vi "RT-Data-in.vi"(2 "cluster":T1, 3 "Amount of Inputs":i32) -> (0 "Error":T1, 1 "Bicep+Triceps":dbl[](array[numeric]))   [LabVIEW 2020]
uses:
  <vilib>/Utility/error.llb/Error Cluster From Error Code.vi
  <vilib>/rvi/errors/niLvFpgaAdjustHostInterfaceError.vi
  <vilib>/rvi/interface/nirviReadWriteControl/nirviReadWriteControl.xnode
  NiFpgaLv.dll
  <vilib>/rvi/interface/Simulation/niFpgaSimulationCallBeginRW.vi
panel:
  in  "Size of Window":i32=240
  out "BicepWindow":dbl[](array[numeric])
  out "TricepWindow":dbl[](array[numeric])
  out "data 5":dbl(graph)
  out "data 4":dbl(graph)
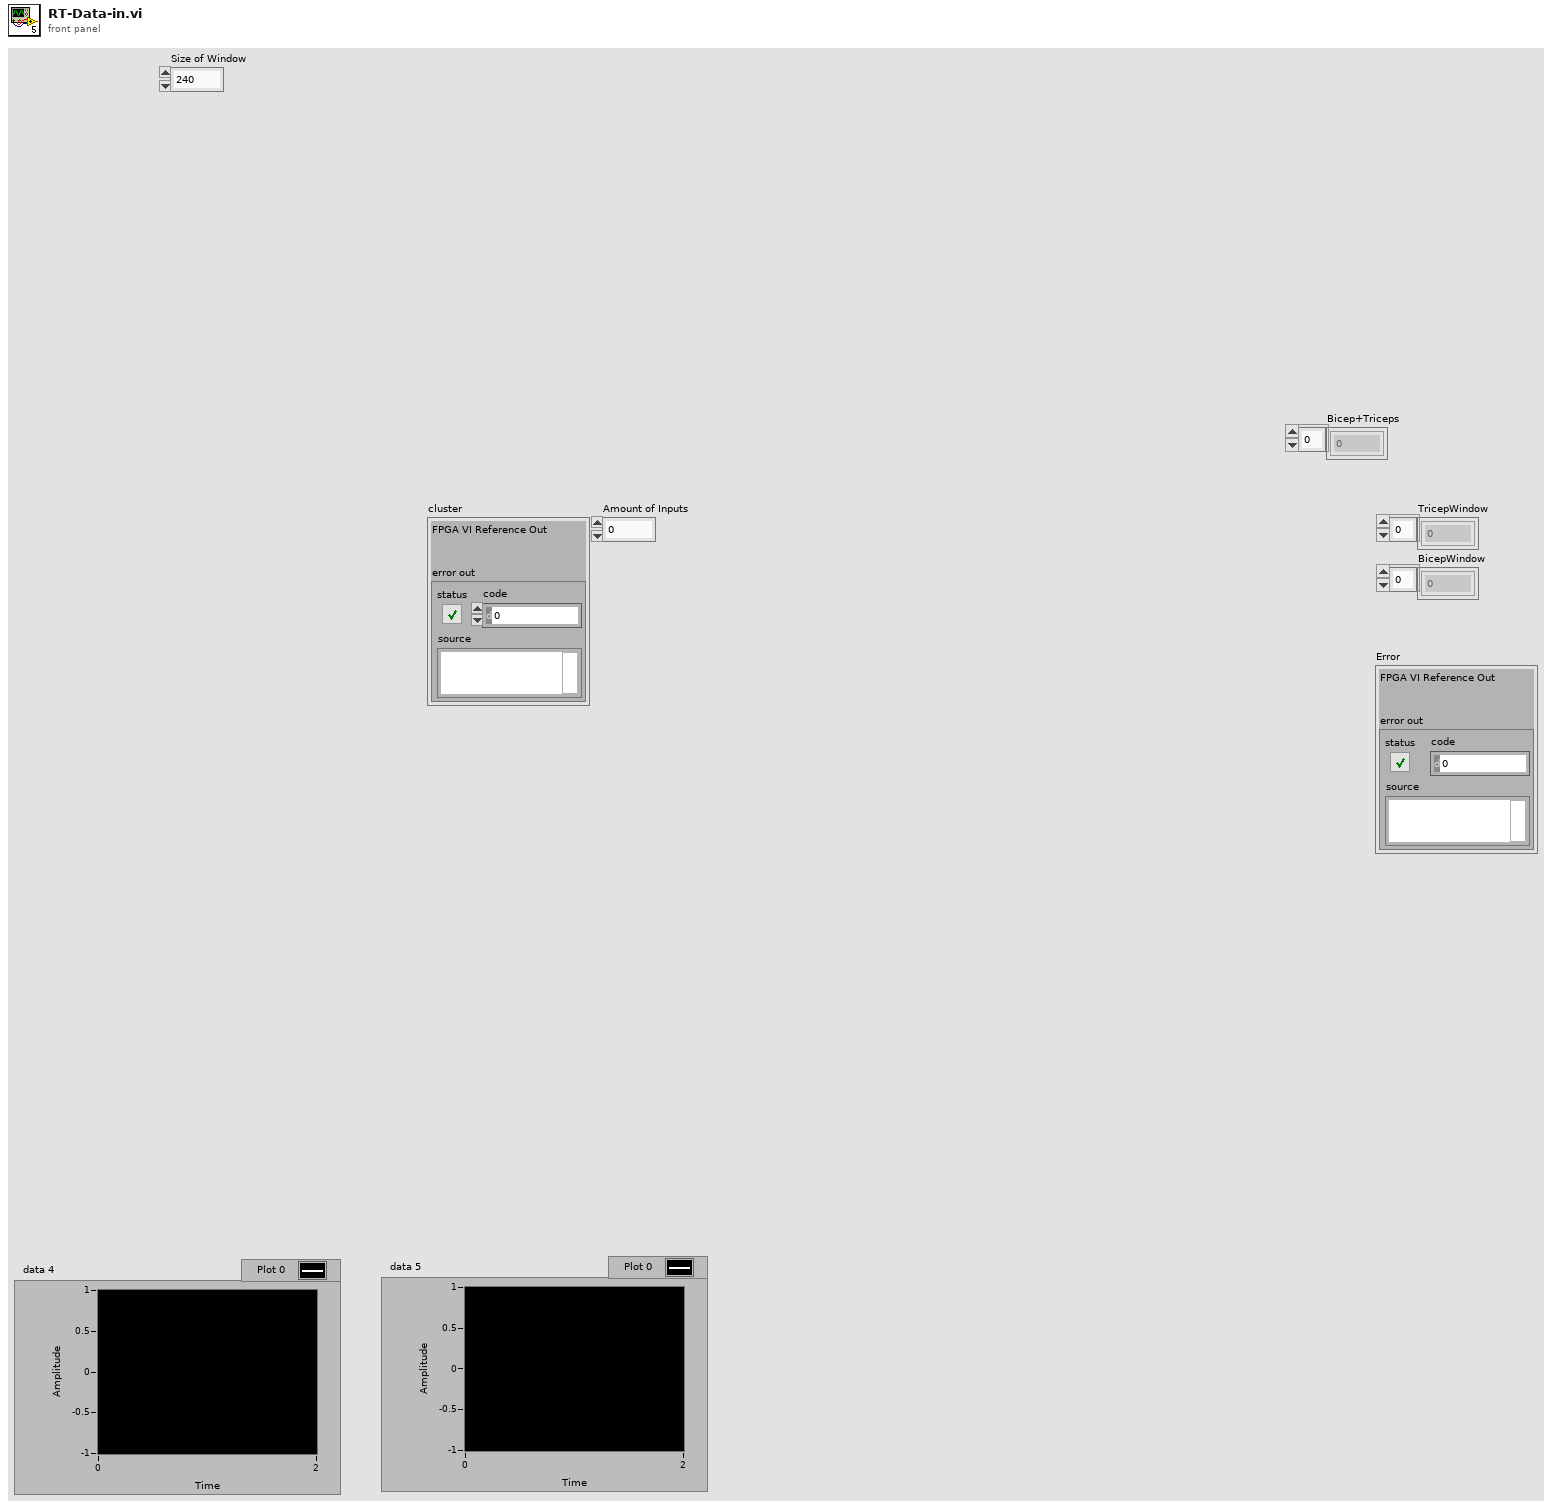
[diagram p1: front panel]
types:
  T1 = cluster{"FPGA VI Reference Out":refnum<k20>, "error out":errorcluster}
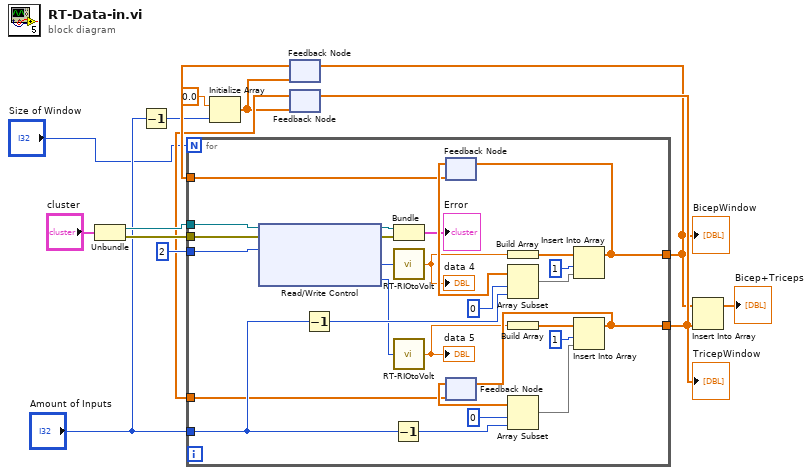
[diagram p0: block diagram]
diagram:
  n1 = Unbundle("cluster") -> ("FPGA VI Reference Out"=w12:refnum<k20>, "error out"=w13:errorcluster)
  n2 = Decrement(x="Amount of Inputs") -> (x-1=w7:i32)
  n3 = Initialize Array(0.0 ("element"), w7) -> (w5:dbl[])
  n4 = feedback #1(w5) -> (w10:dbl[])
  n5 = feedback #2(w5) -> (w9:dbl[])
  n6 = for {
    N: "Size of Window" -> [_]
    tunnel: w13 -> [w41]
    tunnel: w12 -> [w40]
    tunnel: [w34] -> w3
    tunnel: [w26] -> w4
    tunnel: "Amount of Inputs" -> [w25]
    tunnel: i16 2 ("Nr of Analog Inputs") -> [w21]
    tunnel: w10 -> [w20]
    tunnel: w9 -> [w19]
    n7 = xnode ("Read/Write Control")("FPGA VI Reference In"=w40, "error in"=w41, "Nr of Analog Inputs"=w21) -> ("FPGA VI Reference Out"=w22:refnum<k20>, "error out"=w24:errorcluster, "AnalogIn0"=w16:u16, "AnalogIn1"=w18:u16)
    n8 = Decrement(x=w25) -> (x-1=w36:i32)
    n9 = Decrement(x=w25) -> (x-1=w29:i32)
    n10 = Bundle("FPGA VI Reference Out"=w22, "error out"=w24) -> (→"Error":T1)  [unwired: 1 in]
    n11 = call "RT-RIOtoVolt.vi"("Rio-In"=w16) -> ("Volt-Out"=w15:dbl)
    "data 4" <- w15
    n12 = call "RT-RIOtoVolt.vi"("Rio-In"=w18) -> ("Volt-Out"=w17:dbl)
    "data 5" <- w17
    n13 = feedback #3(w20) -> (w38:dbl[])
    n14 = feedback #4(w19) -> (w31:dbl[])
    n15 = Build Array(w15) -> (w27:dbl[])
    n16 = Array Subset(array=w38, index=0, length=w36) -> (w35:dbl[])
    n17 = Build Array(w17) -> (w33:dbl[])
    n18 = Array Subset(array=w31, index=0, length=w29) -> (w28:dbl[])
    n19 = Insert Into Array(array=w27, index=1, new element=w35) -> (w34:dbl[])
    n20 = feedback-in #3(w34) -> ()
    n21 = Insert Into Array(array=w33, index=1, new element=w28) -> (w26:dbl[])
    n22 = feedback-in #4(w26) -> ()
  }
  "TricepWindow" <- w4
  "BicepWindow" <- w3
  n23 = feedback-in #1(w3) -> ()
  n24 = feedback-in #2(w4) -> ()
  n25 = Insert Into Array(array=w3, new element=w4) -> (→"Bicep+Triceps":dbl[])  [unwired: 1 in]
